vi "VI_A.vi"() -> ()   [LabVIEW 2013]
uses:
  stop_A.vi
  stop_B.vi
panel:
  out "lettere che hanno\nfermato VI_B":string[](array[string])
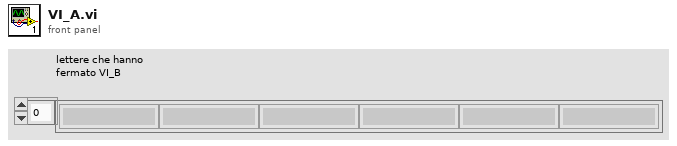
[diagram p1: front panel]
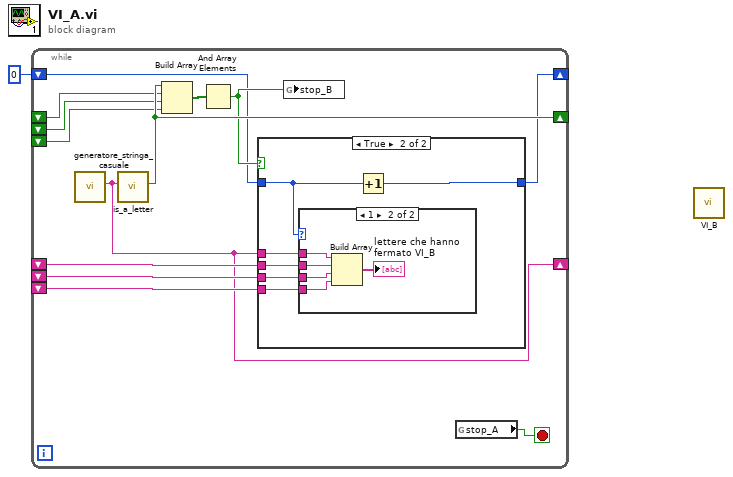
[diagram p0: block diagram]
diagram:
  n1 = while {
    shift-right: [w14] -> _
    shift-left: _ -> [w13]
    shift-left: _ -> [w12]
    shift-left: _ -> [w11]
    shift-right: [w5] -> _
    shift-left: _ -> [w8]
    shift-left: _ -> [w7]
    shift-left: _ -> [w6]
    shift-right: [w3] -> _
    shift-left: 0 -> [w2]
    stop <- w10 stop-if-true
    n2 = call "generatore_stringa_casuale.vi"() -> ("stringa"=w5:string)  [unwired: 11 in]
    n3 = call "is_a_letter.vi"("String"=w5) -> ("is a letter"=w14:bool)  [unwired: 10 in]
    n4 = Build Array(w14, w13, w12, w11) -> (w9:bool[])
    n5 = And Array Elements(Boolean array=w9) -> (logical AND=w4:bool)
    n6 = case shown="True" w4 {
      tunnel: w8 -> [_ w21]
      tunnel: w7 -> [_ w20]
      tunnel: w6 -> [_ w19]
      tunnel: w5 -> [_ w18]
      tunnel: [w15 w16] -> w3
      tunnel: w2 -> [w15 w17]
      frame False {
      }
      frame True {
        n7 = case shown="1" w17 {
          tunnel: w21 -> [_ w26]
          tunnel: w20 -> [_ w25]
          tunnel: w19 -> [_ w24]
          tunnel: w18 -> [_ w23]
          frame 0, Default {
          }
          frame 1 {
            n8 = Build Array(w23, w26, w25, w24) -> (→"lettere che hanno\nfermato VI_B":string[])
          }
        }
        n9 = Increment(x=w17) -> (x+1=w16:i32)
      }
    }
    n10 = global write "stop_B.vi" "stop_B"(w4) -> ()
    n11 = global read "stop_A.vi" "stop_A"() -> (w10:bool)
  }
  n12 = call "VI_B.vi"() -> ()  [unwired: 12 in]
